vi "Add Lookup Event Listener Helper.vi"   [LabVIEW 2019, in "Lookup API.lvlib"]
doc: "This helper includes code to manage type-casting the user event type."
uses:
  Lookup API.lvlib
  605cf116-c6a1-4699-92bc-2b46e486f691.vi
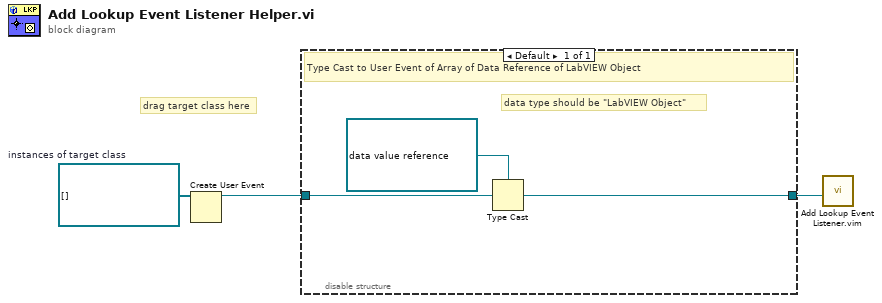
[diagram p0: block diagram]
diagram:
  w3 = refnum<data-value>[] []  # instances of target class
  # "drag target class here"
  n1 = Create User Event(user event datatype=w3) -> (user event=w2:refnum<user-event>)  [unwired: 1 in, 1 out]
  n2 = disable-structure shown="Default" {
    disable-tunnel: w2 -> [w5]
    disable-tunnel: [w4] -> w1
    frame Enabled {
      # "data type should be \"LabVIEW Object\""
      # "Type Cast to User Event of Array of Data Reference of LabVIEW Object"
      n3 = Type Cast(type=refnum<user-event> refnum ("Lookup Listener User Event"), x=w5) -> (*(type *) &x=w4:refnum<user-event>)
    }
  }
  n4 = call "Add Lookup Event Listener.vim"("user event"=w1) -> ()  [unwired: 9 in, 2 out]
